vi "valve_control.vi"(2 "PID Control":T1={"proportional gain (Kc)"=1.0, "integral time (Ti, min)"=0.01, "derivative time (Td, min)"=0.0, "Valve Voltage [V]"=0.0, "Min % Open"=2.0, "Max % Open"=3.0, "Reinitialize?"=FALSE, "Valve On/Off"=FALSE, "Mode"=FALSE, "Full Flow Rate"=0.0, "Flow Set Point [g/s]"=0.0, "AutoTune"=FALSE} {"Flow Set Point [g/s]" format="%.2f"; "Full Flow Rate" format="%.2f"; "Max % Open" min=0.0 max=100.0 format="%.2f"; "Min % Open" min=0.0 max=100.0 format="%.2f"; "Valve Voltage [V]" format="%.2f"; "derivative time (Td, min)" format="%.3f"; "integral time (Ti, min)" format="%.3f"; "proportional gain (Kc)" format="%.3f"}, 3 "Flow rate [g/s]":dbl format="%#_13g") -> (0 "Valve Voltage [V]":dbl, 1 "PID Control Output":T1={"proportional gain (Kc)"=1.0, "integral time (Ti, min)"=0.01, "derivative time (Td, min)"=0.0, "Valve Voltage [V]"=0.0, "Min % Open"=2.0, "Max % Open"=3.0, "Reinitialize?"=FALSE, "Valve On/Off"=FALSE, "Mode"=FALSE, "Full Flow Rate"=0.0, "Flow Set Point [g/s]"=0.0, "AutoTune"=FALSE} {"Flow Set Point [g/s]" format="%.2f"; "Full Flow Rate" format="%.2f"; "Max % Open" min=0.0 max=100.0 format="%.2f"; "Min % Open" min=0.0 max=100.0 format="%.2f"; "Valve Voltage [V]" format="%.2f"; "derivative time (Td, min)" format="%.3f"; "integral time (Ti, min)" format="%.3f"; "proportional gain (Kc)" format="%.3f"})   [LabVIEW 2016]
uses:
  <vilib>/addons/control/pid/NI_PID_autopid.lvlib
  valve_pid_control.ctl
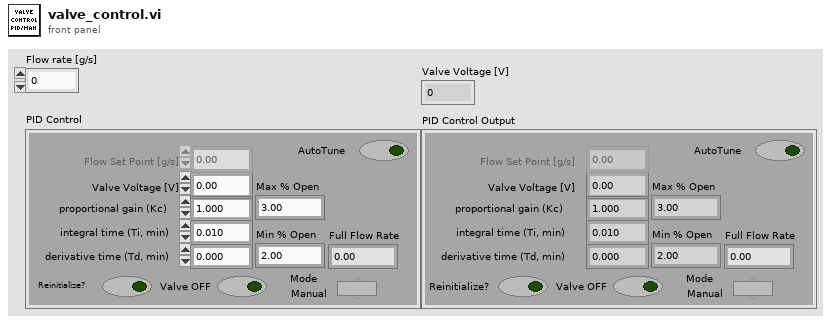
[diagram p1: front panel]
types:
  T1 = typedef "valve_pid_control.ctl" = cluster{"proportional gain (Kc)":dbl, "integral time (Ti, min)":dbl, "derivative time (Td, min)":dbl, "Valve Voltage [V]":dbl, "Min % Open":dbl, "Max % Open":dbl, "Reinitialize?":bool, "Valve On/Off":bool, "Mode":bool, "Full Flow Rate":dbl, "Flow Set Point [g/s]":dbl, "AutoTune":bool}
  T2 = cluster{"proportional gain (Kc)":dbl, "integral time (Ti, min)":dbl, "derivative time (Td, min)":dbl}
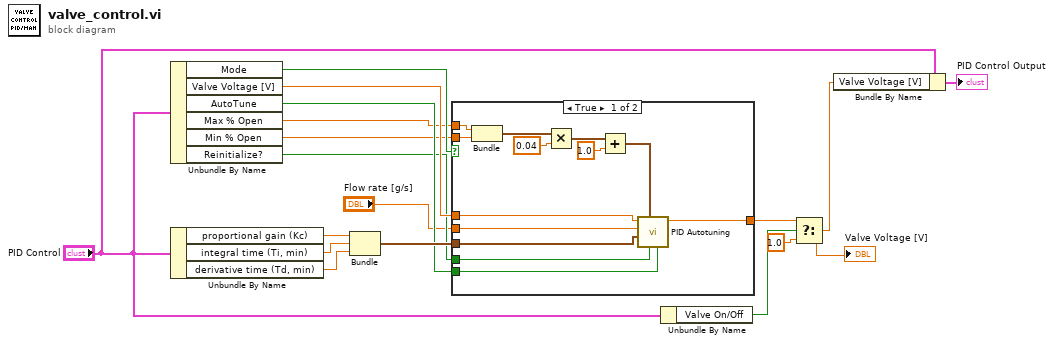
[diagram p0: block diagram]
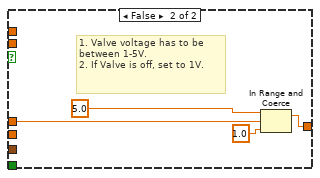
[diagram p2: hidden frame]
diagram:
  n1 = Unbundle By Name("PID Control") -> ("Mode"=w17:bool, "Valve Voltage [V]"=w14:dbl, "AutoTune"=w15:bool, "Max % Open"=w8:dbl, "Min % Open"=w7:dbl, "Reinitialize?"=w13:bool)
  n2 = Unbundle By Name("PID Control") -> ("proportional gain (Kc)"=w11:dbl, "integral time (Ti, min)"=w10:dbl, "derivative time (Td, min)"=w9:dbl)
  n3 = Bundle("proportional gain (Kc)"=w11, "integral time (Ti, min)"=w10, "derivative time (Td, min)"=w9) -> (w16:T2)  [unwired: 1 in]
  n4 = case shown="True" w17 {
    tunnel: [w24 w31] -> w3
    tunnel: w14 -> [w30 w32]
    tunnel: "Flow rate [g/s]" -> [w29 _]
    tunnel: w16 -> [w28 _]
    tunnel: w13 -> [w27 _]
    tunnel: w8 -> [w26 _]
    tunnel: w7 -> [w25 _]
    tunnel: w15 -> [w23 _]
    frame True {
      n5 = Bundle("Max % Open"=w26, "Min % Open"=w25) -> (w19:cluster{"Max % Open":dbl, "Min % Open":dbl})  [unwired: 1 in]
      n6 = Multiply(x=w19, y=0.04) -> (x*y=w20:cluster{"Max % Open":dbl, "Min % Open":dbl})
      n7 = Add(x=w20, y=1.0) -> (x+y=w21:cluster{"Max % Open":dbl, "Min % Open":dbl})
      n8 = call <vilib>:"PID Autotuning.vi"("autotune? (F)"=w23, "reinitialize? (F)"=w27, "output range"=w21, "PID gains"=w28, "process variable"=w29, "setpoint"=w30) -> ("output"=w24:dbl)  [unwired: 2 in, 3 out]
    }
    frame False {
      # "1. Valve voltage has to be between 1-5V.\n2. If Valve is off, set to 1V."
      n9 = In Range and Coerce(upper limit=5.0, x=w32, lower limit=1.0) -> (coerced(x)=w31:dbl)  [unwired: 1 out]
    }
  }
  n10 = Unbundle By Name("PID Control") -> ("Valve On/Off"=w2:bool)
  n11 = Select(t=w3, s=w2, f=1.0) -> (s? t:f=w1:dbl)
  "Valve Voltage [V]" <- w1
  n12 = Bundle By Name(cluster="PID Control", "Valve Voltage [V]"=w1) -> (→"PID Control Output":T1)
